vi "asap_calibration.vi"() -> ()   [LabVIEW 2012]
uses:
  <vilib>/Utility/file.llb/Read From Spreadsheet File (DBL).vi
panel:
  in  "Settling time":dbl=1.0
  out "Out OK":bool
  out "In OK":bool
  in  "Run":bool
  in  "Input mode":enum16{"Absolute axis", "Relative axis", "Pose"}(ring)=enum."Pose"
  out "Points done":i32
  out "# Points":i32
  out "Position":dbl[](array[numeric]) format="%#_3p"
  out "State":enum16{"Initialize", "Move", "Log", "Done"}(ring)
  in  "Axis names":string[](array[string])=["X", "Y", "Z", "Rx", "Ry", "Rz"]
  in  "Axis enable":bool[](array[boolean])=[TRUE, TRUE, TRUE, TRUE, TRUE, TRUE]
  in  "stop":bool
  in  "Point time":dbl=1.0
  out "ASAP status":cluster{"Valid position":bool, "Message":string}
  in  "Output file":path=path "C:/Users/ram/Documents/work/Micron/asap/cal_data/SN1/sensor_cal/sensor_cal.dat"
  in  "Input points file":path=path "C:/Users/ram/Documents/work/Micron/asap/matlab/psd_cal.dat"
  # "ASAP calibration motion controller"
  # "Point"
  # "of"
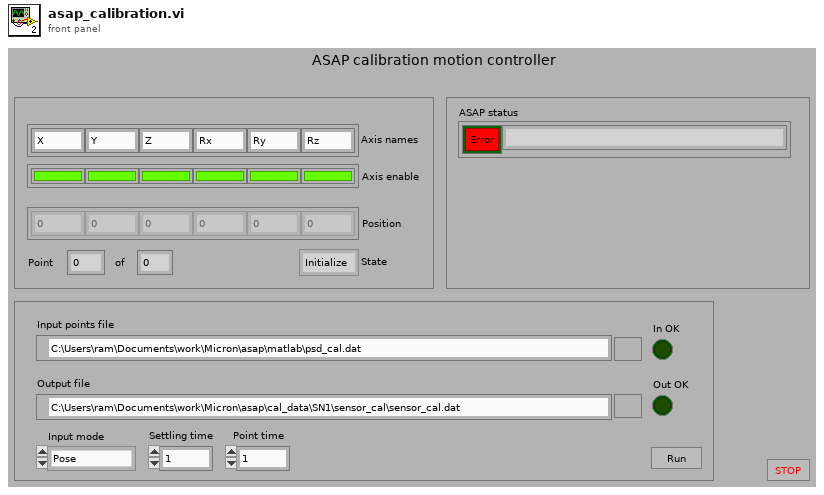
[diagram p1: front panel]
types:
  T1 = enum16{"open", "replace", "create", "open or create", "replace or create", "replace or create with confirmation"}
  T2 = typedef "motion_status.ctl" = cluster{"Axis names":string[], "Axis positions":dbl[], "Pose":dbl[], "Timestamp":u32, "Ready":bool, "Stopped":bool}
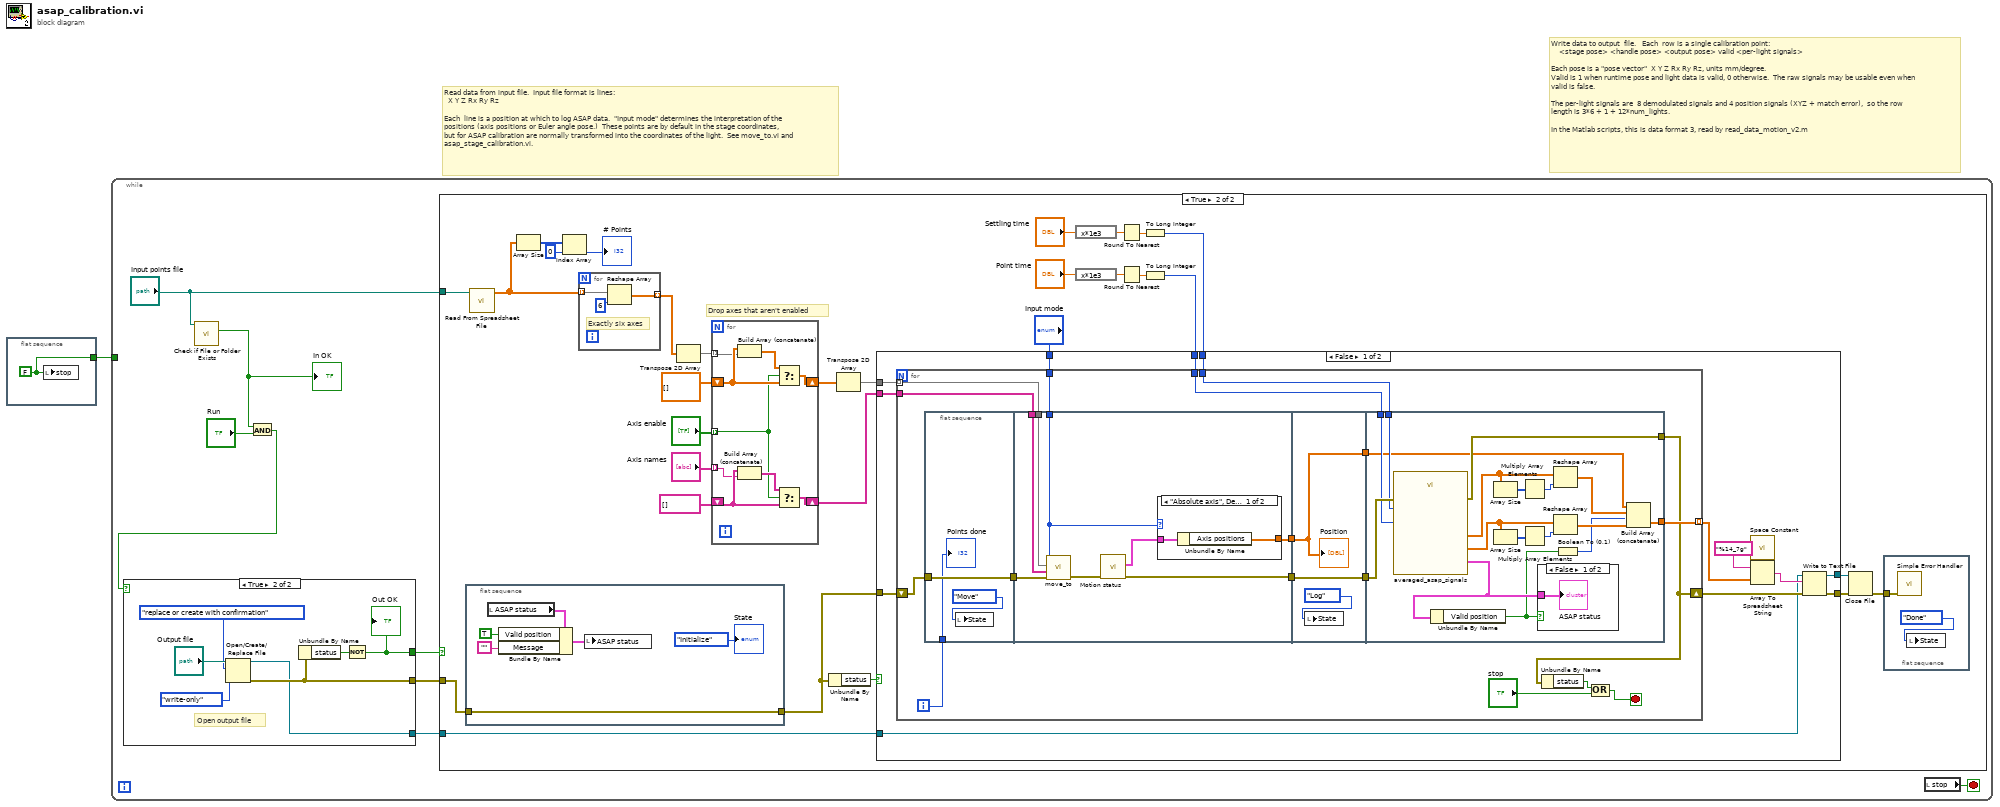
[diagram p0: block diagram]
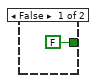
[diagram p2: hidden frame]
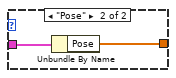
[diagram p4: hidden frame]
diagram:
  # "Write data to output  file.   Each  row is a single calibration point:\n    <stage pose> <handle pose> <output pose> valid <per-light signals>\n\nEach pose is a \"pose vector\"  X Y Z Rx Ry Rz, units mm/degree.\nValid is 1 when runtime pose and light data is valid, 0 otherwise.  The raw signals may be usable even when valid is false.\n\nThe per-light signals are  8 demodulated signals and 4 position signals (XYZ + match error),  so the row length is 3*6 + 1 + 12*num_lights.\n\nIn the Matlab scripts, this is data format 3, read by read_data_motion_v2.m"
  # "Read data from input file.  Input file format is lines:\n  X Y Z Rx Ry Rz\n\nEach  line is a position at which to log ASAP data.  \"Input mode\" determines the interpretation of the positions (axis positions or Euler angle pose.)  These points are by default in the stage coordinates, but for ASAP calibration are normally transformed into the coordinates of the light.  See move_to.vi and asap_stage_calibration.vi."
  n1 = flat-sequence {
    tunnel: [w2] -> w1
    frame #0 {
      w2 = FALSE ("stop")
      n2 = local write "stop"(w2) -> ()
    }
  }
  n3 = while {
    tunnel: w1 -> [_]
    stop <- w7 stop-if-true
    n4 = call <vilib>:"Check if File or Folder Exists.vi"("path"="Input points file") -> ("file or folder exists?"=w3:bool)  [unwired: 8 in, 2 out]
    "In OK" <- w3
    n5 = And(x=w3, y="Run") -> (x .and. y?=w5:bool)
    n6 = case shown="True" w5 {
      tunnel: [_ w18] -> w9
      tunnel: [_ w17] -> w8
      tunnel: [FALSE w12] -> w4
      frame False {
      }
      frame True {
        # "Open output file"
        n7 = Open/Create/Replace File(file path (use dialog)="Output file", operation (0:open)=T1."replace or create with confirmation", access (0:read/write)=enum16{"read/write", "read-only", "write-only"}."write-only") -> (refnum out=w17:refnum<file>, error out=w18:errorcluster)  [unwired: 3 in, 1 out]
        n8 = Unbundle By Name(w18) -> ("status"=w16:bool)
        n9 = Not(x=w16) -> (.not. x?=w12:bool)
        "Out OK" <- w12
      }
    }
    n10 = case shown="True" w4 {
      tunnel: "Input points file" -> [_ w47]
      tunnel: w9 -> [_ w31]
      tunnel: w8 -> [_ w33]
      frame False {
      }
      frame True {
        # "Drop axes that aren't enabled"
        n11 = flat-sequence {
          tunnel: w31 -> [w57]
          tunnel: [w57] -> w30
          frame #0 {
            n12 = local read "ASAP status"() -> (w53:cluster{"Valid position":bool, "Message":string})
            n13 = Bundle By Name(cluster=w53, "Valid position"=TRUE, "Message"="") -> (w55:cluster{"Valid position":bool, "Message":string})
            n14 = local write "ASAP status"(w55) -> ()
            "State" <- enum16{"Initialize", "Move", "Log", "Done"}."Initialize" ("State")
          }
        }
        n15 = call-poly <vilib>:"Read From Spreadsheet File.vi"("file path (dialog if empty)"=w47) -> ("all rows"=w29:dbl[][])  [unwired: 6 in, 4 out]
        n16 = Array Size(array=w29) -> (size(s)=w36:i32[])
        n17 = Index Array(array=w36, index=0) -> (element=→"# Points":i32)
        n18 = for {
          tunnel: w29 -> [w51] mode=indexing
          tunnel: [w49] -> w27 mode=indexing
          # "Exactly six axes"
          n19 = Reshape Array(w51, 6 ("dimension size")) -> (w49:dbl[])
        }
        n20 = Transpose 2D Array(2D array=w27) -> (transposed array=w41:dbl[][])
        n21 = for {
          shift-right: [w65] -> w35
          shift-left: dbl[][] [] ("all rows") -> [w68]
          tunnel: "Axis enable" -> [w60] mode=indexing
          tunnel: w41 -> [w67] mode=indexing
          shift-right: [w61] -> w38
          shift-left: string[] [] ("Axis names") -> [w63]
          tunnel: "Axis names" -> [w62] mode=indexing
          n22 = Build Array (concatenate)(w68, w67) -> (w66:dbl[][])
          n23 = Build Array (concatenate)(w63, w62) -> (w64:string[])
          n24 = Select(t=w66, s=w60, f=w68) -> (s? t:f=w65:dbl[][])
          n25 = Select(t=w64, s=w60, f=w63) -> (s? t:f=w61:string[])
        }
        n26 = Unbundle By Name(w30) -> ("status"=w48:bool)
        n27 = Transpose 2D Array(2D array=w35) -> (transposed array=w34:dbl[][])
        n28 = expression code="x*1e3"("Settling time") -> (w21:dbl)
        n29 = expression code="x*1e3"("Point time") -> (w25:dbl)
        n30 = Round To Nearest(number=w21) -> (nearest integer value=w22:dbl)
        n31 = Round To Nearest(number=w25) -> (nearest integer value=w24:dbl)
        n32 = To Long Integer(number=w22) -> (32bit integer=w19:i32)
        n33 = To Long Integer(number=w24) -> (32bit integer=w23:i32)
        n34 = case shown="False" w48 {
          tunnel: w30 -> [w76 w136]
          tunnel: w33 -> [w75 w137]
          tunnel: w34 -> [w82 _]
          tunnel: [w79 w137] -> w46
          tunnel: [w77 w136] -> w45
          tunnel: w38 -> [w74 _]
          tunnel: "Input mode" -> [w73 _]
          tunnel: w23 -> [w71 _]
          tunnel: w19 -> [w70 _]
          frame False {
            n35 = for {
              tunnel: w82 -> [w91] mode=indexing
              tunnel: [w99] -> w72 mode=indexing
              shift-right: [w90] -> w78
              shift-left: w76 -> [w98]
              tunnel: w74 -> [w93]
              tunnel: w73 -> [w88]
              tunnel: w71 -> [w86]
              tunnel: w70 -> [w85]
              i -> [w89]
              stop <- w87 stop-if-true
              n36 = flat-sequence {
                tunnel: w98 -> [w102]
                tunnel: [w102] -> w95
                tunnel: w89 -> [w100]
                tunnel: w95 -> [w110]
                tunnel: [w106] -> w94
                tunnel: w93 -> [w109]
                tunnel: w91 -> [w108]
                tunnel: w88 -> [w105]
                tunnel: [w103] -> w84
                tunnel: w94 -> [w117]
                tunnel: [w117] -> w92
                tunnel: w84 -> [w115]
                tunnel: [w115] -> w83
                tunnel: [w133] -> w99
                tunnel: w92 -> [w131]
                tunnel: [w134] -> w90
                tunnel: w86 -> [w126]
                tunnel: w85 -> [w125]
                tunnel: w83 -> [w119]
                frame #0 {
                  n37 = local write "State"(enum16{"Initialize", "Move", "Log", "Done"}."Move" ("State")) -> ()
                  "Points done" <- w100
                }
                frame #1 {
                  n38 = call "move_to.vi"("Error in"=w110, "Axis names"=w109, "Axis positions"=w108, "Mode"=w105) -> ("Error out"=w107:errorcluster)  [unwired: 7 in]
                  n39 = call "Motion status.vi"("error in"=w107) -> ("error out"=w106:errorcluster, "Motion status"=w104:T2)  [unwired: 5 in, 4 out]
                  n40 = case shown="\"Absolute axis\", Default" w105 {
                    tunnel: w104 -> [w112 w114]
                    tunnel: [w111 w113] -> w103
                    frame "Absolute axis", Default {
                      n41 = Unbundle By Name(w112) -> ("Axis positions"=w111:dbl[])
                    }
                    frame "Pose" {
                      n42 = Unbundle By Name(w114) -> ("Pose"=w113:dbl[])
                    }
                  }
                }
                frame #2 {
                  n43 = local write "State"(enum16{"Initialize", "Move", "Log", "Done"}."Log" ("State")) -> ()
                  "Position" <- w115
                }
                frame #3 {
                  n44 = call "averaged_asap_signals.vi"("error in"=w131, "Averaging time (ms)"=w126, "Settling time (ms)"=w125) -> ("error out"=w134:errorcluster, "ASAP diagnostics"=w132:cluster{"Valid position":bool, "Message":string}, "Poses"=w118:sgl[][], "Demodulated averaged"=w128:sgl[][])  [unwired: 5 in]
                  n45 = Unbundle By Name(w132) -> ("Valid position"=w124:bool)
                  n46 = Array Size(array=w118) -> (size(s)=w121:i32[])
                  n47 = Array Size(array=w128) -> (size(s)=w130:i32[])
                  n48 = Multiply Array Elements(1:w121) -> (0:w122:i32)
                  n49 = Multiply Array Elements(1:w130) -> (0:w129:i32)
                  n50 = case shown="False" w124 {
                    tunnel: w132 -> [w135 _]
                    frame False {
                      "ASAP status" <- w135
                    }
                    frame True {
                    }
                  }
                  n51 = Reshape Array(w118, w122) -> (w120:sgl[])
                  n52 = Reshape Array(w128, w129) -> (w127:sgl[])
                  n53 = Boolean To (0,1)(Boolean=w124) -> (0, 1=w123:i16)
                  n54 = Build Array (concatenate)(w119, w120, w123, w127) -> (w133:dbl[])
                }
              }
              n55 = Unbundle By Name(w90) -> ("status"=w97:bool)
              n56 = Compound Arithmetic op=OR(w97, "stop") -> (w87:bool)
            }
            n57 = call <vilib>:"Space Constant.vi"() -> ("String"=w69:string)
            n58 = Array To Spreadsheet String(delimiter (Tab)=w69, array=w72, 3:"%14_7g" ("format (%.3f)")) -> (spreadsheet string=w80:string)
            n59 = Write to Text File(file (use dialog)=w75, text=w80, error in=w78) -> (refnum out=w79:refnum<file>, error out=w77:errorcluster)  [unwired: 1 in, 1 out]
          }
          frame True {
          }
        }
        n60 = Close File(refnum=w46, error in=w45) -> (error out=w44:errorcluster)  [unwired: 1 out]
        n61 = flat-sequence {
          tunnel: w44 -> [w59]
          frame #0 {
            n62 = call <vilib>:"Simple Error Handler.vi"("error in (no error)"=w59) -> ()  [unwired: 4 in, 5 out]
            n63 = local write "State"(enum16{"Initialize", "Move", "Log", "Done"}."Done" ("State")) -> ()
          }
        }
      }
    }
    n64 = local read "stop"() -> (w7:bool)
  }
